vi "Test Decompose and Recompose.vi"() -> ()   [LabVIEW 2018, in "Resource Manipulation.lvlib"]
uses:
  Resource Manipulation.lvlib
  Resource.ctl
  Decompose VI (Path).vi
panel:
  out "Target path out":path
  out "VI Load Result":errorcluster
  out "array of clusters":T2(array[cluster])
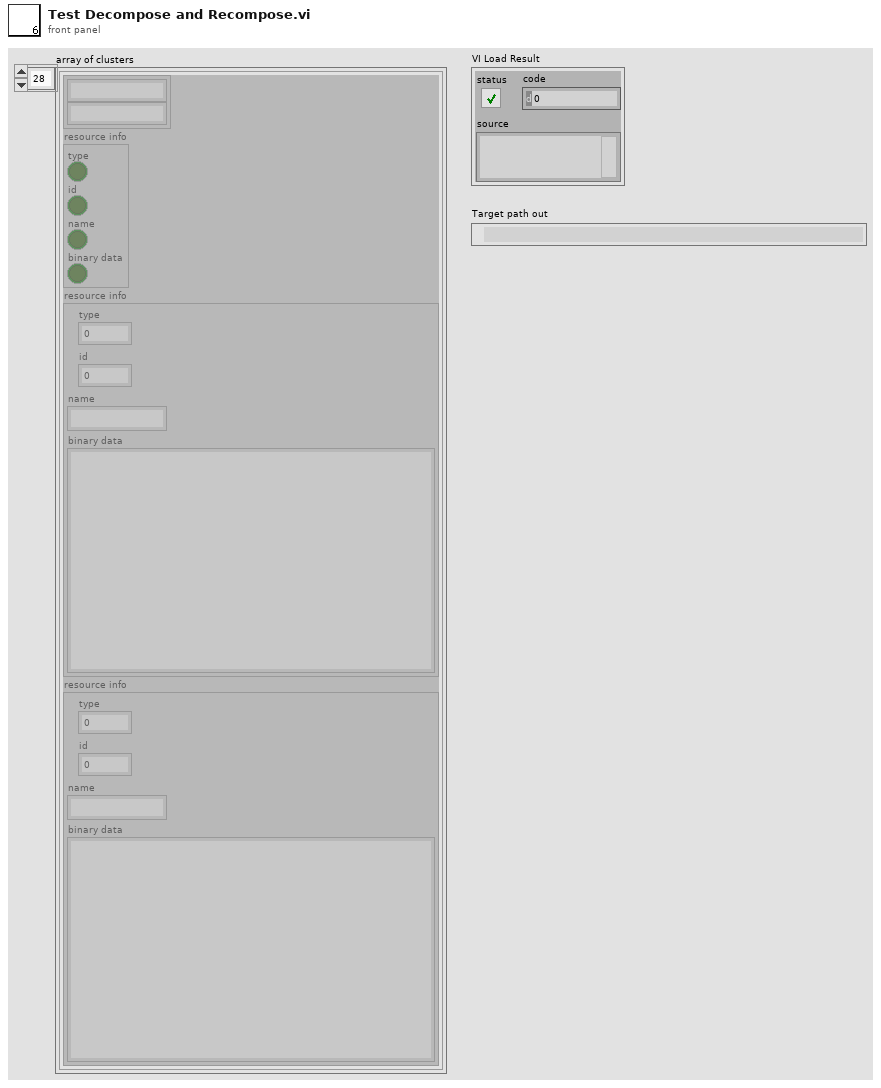
[diagram p1: front panel]
types:
  T1 = typedef "Resource Manipulation.lvlib/Resource.ctl" = cluster{"type":u32, "id":i32, "name":string, "binary data":string}
  T2 = cluster{cluster{string, string}, "resource info":cluster{"type":bool, "id":bool, "name":bool, "binary data":bool}, "resource info":T1, "resource info":T1}[]
  T3 = typedef "Resource Manipulation.lvlib/Resource Array.ctl" = T1[]
  T4 = cluster{"type":bool, "id":bool, "name":bool, "binary data":bool}[]
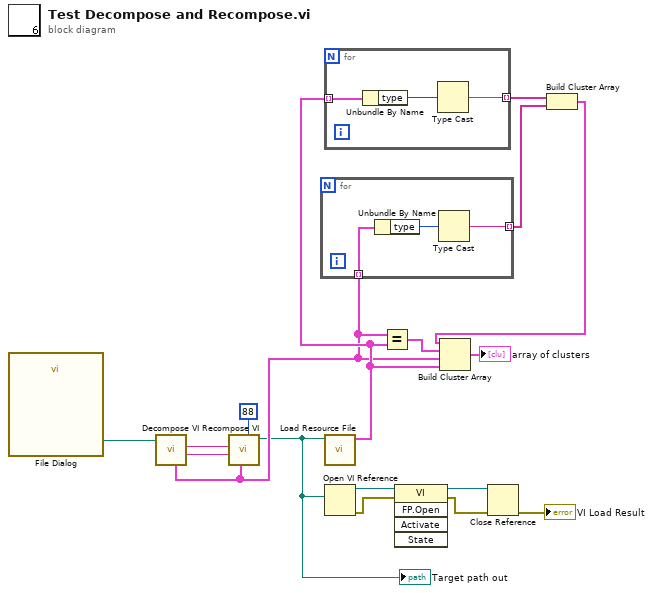
[diagram p0: block diagram]
diagram:
  n1 = call "File Dialog"() -> ("selected path"=w15:path)  [unwired: 12 in, 3 out]
  n2 = call-poly "Decompose VI.vi"("VI path"=w15) -> ("Block Diagram XML"=w17:string, "Front Panel XML"=w1:string, "Other resources"=w8:T3)  [unwired: 6 in, 2 out]
  n3 = call "Recompose VI.vi"("FPH_/BDH_ (88=X)"=u8 88, "Other resources (default)"=w8, "Block Diagram XML"=w17, "Front Panel XML"=w1) -> ("Target path out"=w7:path)  [unwired: 5 in, 2 out]
  "Target path out" <- w7
  n4 = for {
    tunnel: w8 -> [w20] mode=indexing
    tunnel: [w18] -> w11 mode=indexing
    n5 = Unbundle By Name(w20) -> ("type"=w19:u32)
    n6 = Type Cast(x=w19) -> (*(type *) &x=w18:string)  [unwired: 1 in]
  }
  n7 = call "Load Resource File.vi"("Resource file"=w7) -> ("Resources"=w13:T3)  [unwired: 8 in, 2 out]
  n8 = for {
    tunnel: w13 -> [w23] mode=indexing
    tunnel: [w21] -> w12 mode=indexing
    n9 = Unbundle By Name(w23) -> ("type"=w22:u32)
    n10 = Type Cast(x=w22) -> (*(type *) &x=w21:string)  [unwired: 1 in]
  }
  n11 = Open VI Reference(vi path=w7) -> (vi reference=w6:refnum<vi>, error out=w5:errorcluster)  [unwired: 5 in]
  n12 = Equal?(x=w8, y=w13) -> (x = y?=w14:T4)
  n13 = invoke class="VI" method="FP.Open"(reference=w6, error in=w5) -> (reference out=w4:refnum<vi>, error out=w3:errorcluster)  [unwired: 3 in, 3 out]
  n14 = Close Reference(reference=w4, error in (no error)=w3) -> (error out=→"VI Load Result":errorcluster)
  n15 = Build Cluster Array(w12, w11) -> (w10:cluster{string, string}[])
  n16 = Build Cluster Array(w10, w14, w8, w13) -> (→"array of clusters":T2)
